vi "Create_LV_INI_Token.vi"   [LabVIEW 2020]
uses:
  <vilib>/Wiresmith Technology/G CLI/CLI Class/CLI.lvclass
  <vilib>/Utility/config.llb/NI_LVConfig.lvlib
  <vilib>/Utility/config.llb/Write Key (String).vi
types:
  T1 = enum32{"Invalid", "Standard", "Closed", "Hidden", "Minimized", "Maximized"}
  T2 = typedef "NI_LVConfig.lvlib/Config Data RefNum.ctl" = refnum<k1>
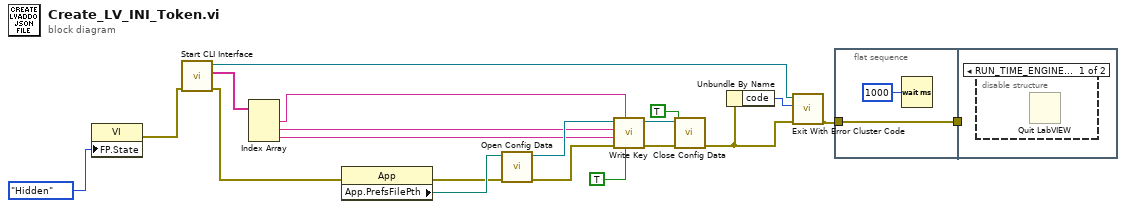
[diagram p0: block diagram]
diagram:
  n1 = property class="VI"("FP.State"=T1."Hidden" ("Front Panel Window:State")) -> (error out=w19:errorcluster)  [unwired: 2 in, 1 out]
  n2 = call <vilib>:"Start CLI Interface.vi"("error in (no error)"=w19) -> ("error out"=w10:errorcluster, "Custom Parameters"=w11:string[], "CLI out"=w18:refnum<class "CLI.lvclass">)  [unwired: 7 in, 1 out]
  n3 = Index Array(array=w11) -> (element #1=w7:string, element #2=w6:string, element #3=w5:string)  [unwired: 3 in]
  n4 = property class="App"(error in=w10) -> (error out=w14:errorcluster, "App.PrefsFilePth"=w17:path)  [unwired: 1 in, 1 out]
  n5 = call <vilib>:"Open Config Data.vi"("error in (no error)"=w14, "configuration file path"=w17) -> ("error out"=w15:errorcluster, "refnum"=w16:T2)  [unwired: 7 in, 1 out]
  n6 = call-poly <vilib>:"Write Key.vi"("write raw string? (F)"=TRUE, "section"=w7, "error in (no error)"=w15, "value"=w5, "key"=w6, "refnum"=w16) -> ("error out"=w13:errorcluster, "refnum out"=w12:T2)  [unwired: 3 in, 1 out]
  n7 = call <vilib>:"Close Config Data.vi"("error in (no error)"=w13, "write file if changed (T)"=TRUE, "refnum"=w12) -> ("error out"=w4:errorcluster)  [unwired: 7 in, 1 out]
  n8 = Unbundle By Name(w4) -> ("code"=w3:i32)
  n9 = call <vilib>:"Exit With Error Cluster Code.vi"("error in (no error)"=w4, "No Error Code (0)"=w3, "CLI in"=w18) -> ("error out"=w1:errorcluster)  [unwired: 8 in]
  n10 = flat-sequence {
    tunnel: w1 -> [w22]
    tunnel: [w22] -> w2
    tunnel: w2 -> [_]
    frame #0 {
      n11 = Wait (ms)(milliseconds to wait=u32 1000) -> ()  [unwired: 1 out]
    }
    frame #1 {
      n12 = disable-structure shown="RUN_TIME_ENGINE==True" {
        frame condition #0 {
          n13 = Quit LabVIEW() -> ()  [unwired: 1 in]
        }
        frame condition #1 (active) {
        }
      }
    }
  }
